vi "Get Description.vi"(8 "error in (no error)":errorcluster, 10 "Tag":string, 11 "Test Tree In":refnum<class "Test Tree.lvclass">) -> (0 "error out":errorcluster, 1 "found?":bool, 2 "Description":string, 3 "Test Tree Out":refnum<class "Test Tree.lvclass">)   [LabVIEW 2020, in "Test Tree.lvclass"]
uses:
  Test Tree.lvclass
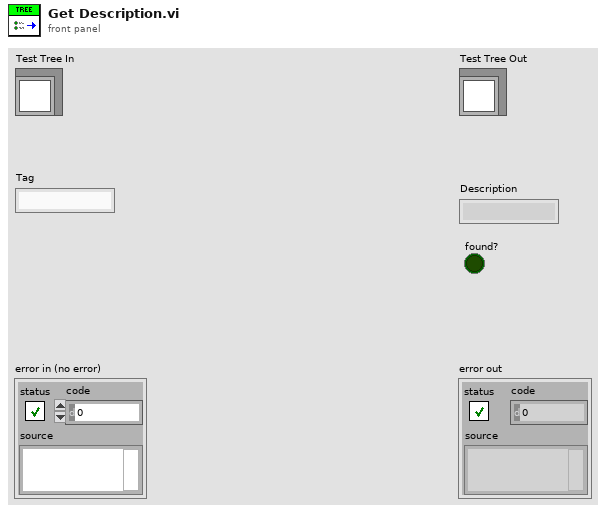
[diagram p1: front panel]
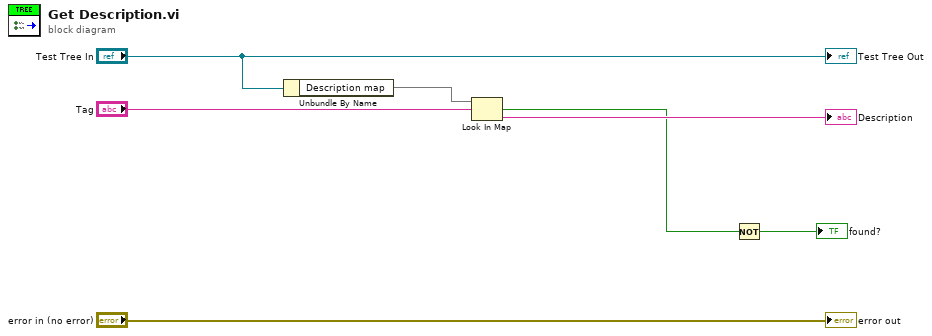
[diagram p0: block diagram]
diagram:
  n1 = Unbundle By Name("Test Tree In") -> ("Description map"=w5:map{string, string})
  n2 = Look In Map(map=w5, key="Tag") -> (key not found?=w2:bool, value=→"Description":string)  [unwired: 1 in]
  n3 = Not(x=w2) -> (.not. x?=→"found?":bool)
  "error out" <- "error in (no error)"
  "Test Tree Out" <- "Test Tree In"
